vi "Refresh Item (inline).vi"(8 "error in (no error)":errorcluster, 10 "Item Index":i32, 11 "BetterHandle in":refnum<class "BetterHandle.lvclass">) -> (0 "error out":errorcluster, 3 "BetterHandle out":refnum<class "BetterHandle.lvclass">)   [LabVIEW 2020, in "BetterDragAndDrop.lvlib" / "BetterHandle.lvclass"]
uses:
  BetterHandle.lvclass
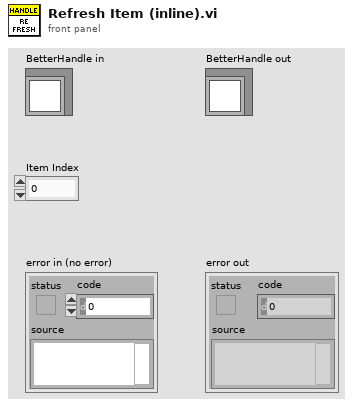
[diagram p1: front panel]
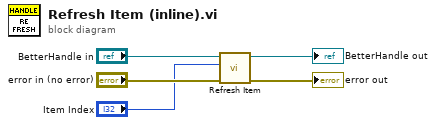
[diagram p0: block diagram]
diagram:
  n1 = call-dynamic "Refresh Item.vi"("error in (no error)"="error in (no error)", "Item Index"="Item Index", "BetterHandle in"="BetterHandle in") -> ("error out"=→"error out":errorcluster, "BetterHandle out"=→"BetterHandle out":refnum<class "BetterHandle.lvclass">)  [unwired: 7 in]
